vi "读取反控数据解析(子VI).vi"(6 "数据":string, 7 "命令编码CN":string) -> (0 "实时数据发送时间间隔/min":i32=1, 2 "设置超时时间/min":i32=1, 3 "反控命令错误？":bool)   [LabVIEW 2016, in "数据传输系统.lvlib"]
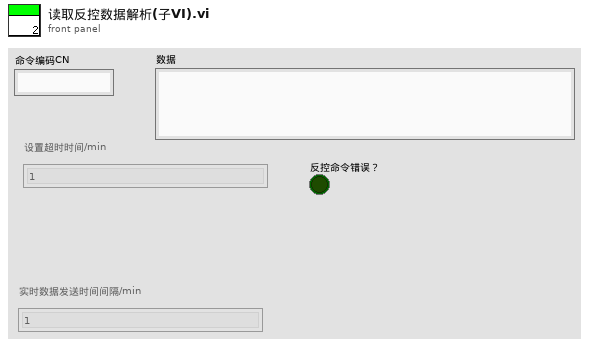
[diagram p1: front panel]
types:
  T1 = enum16{"初始化", "打开连接", "表格比对", "发送数据", "读取数据", "数据处理"}
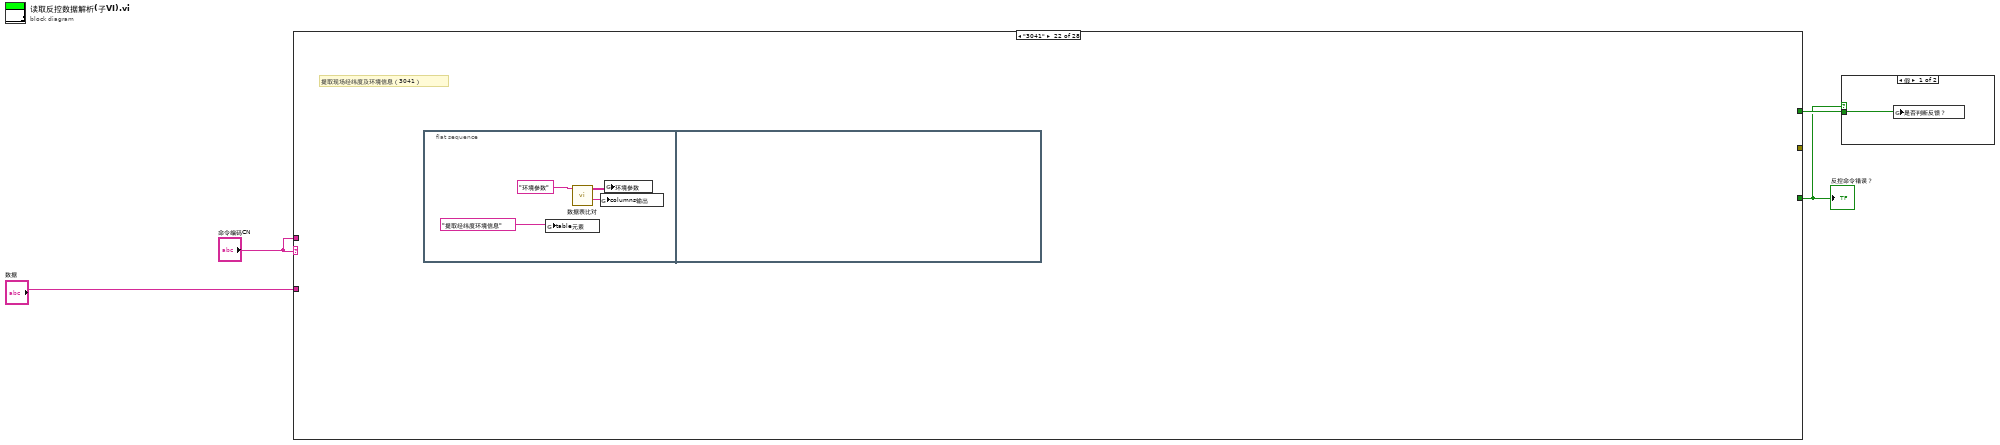
[diagram p0: block diagram]
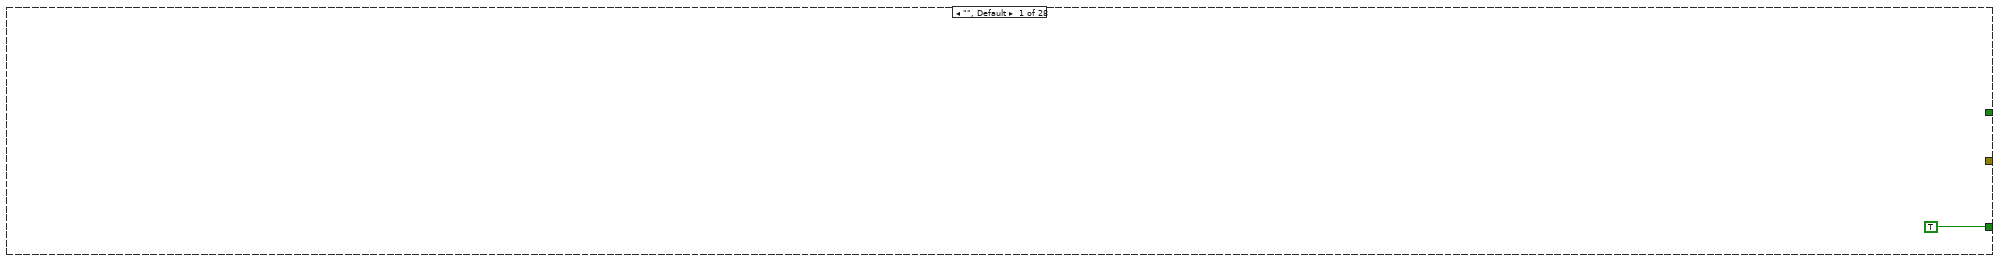
[diagram p3: hidden frame]
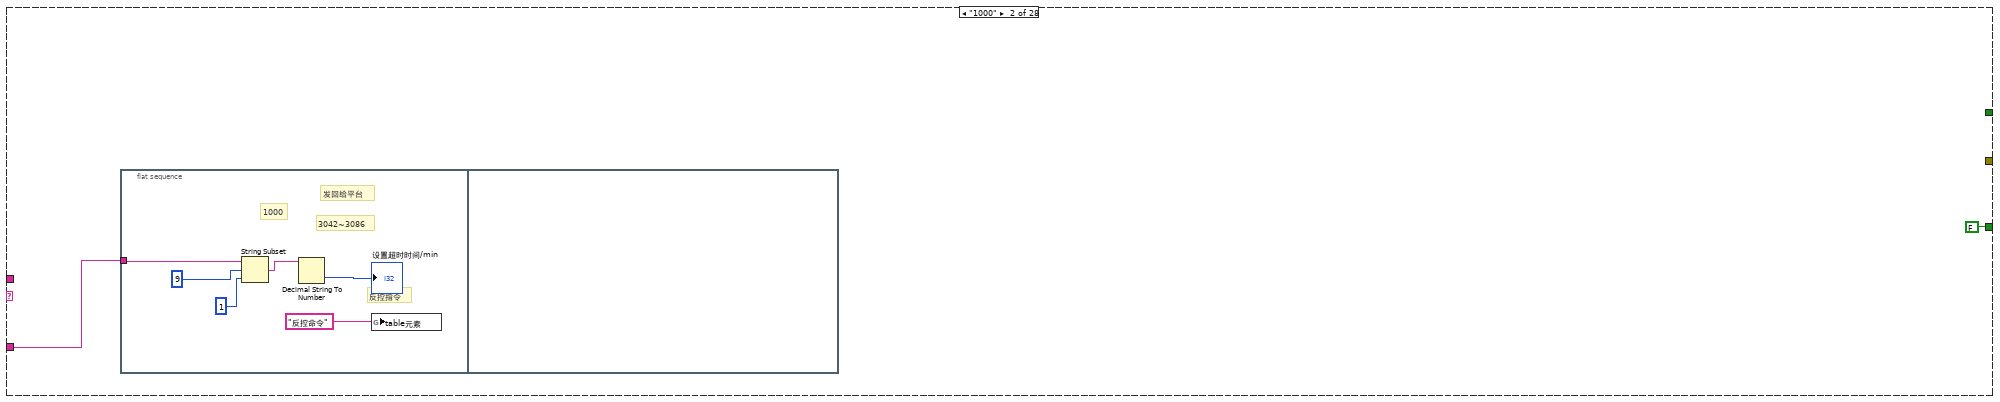
[diagram p4: hidden frame]
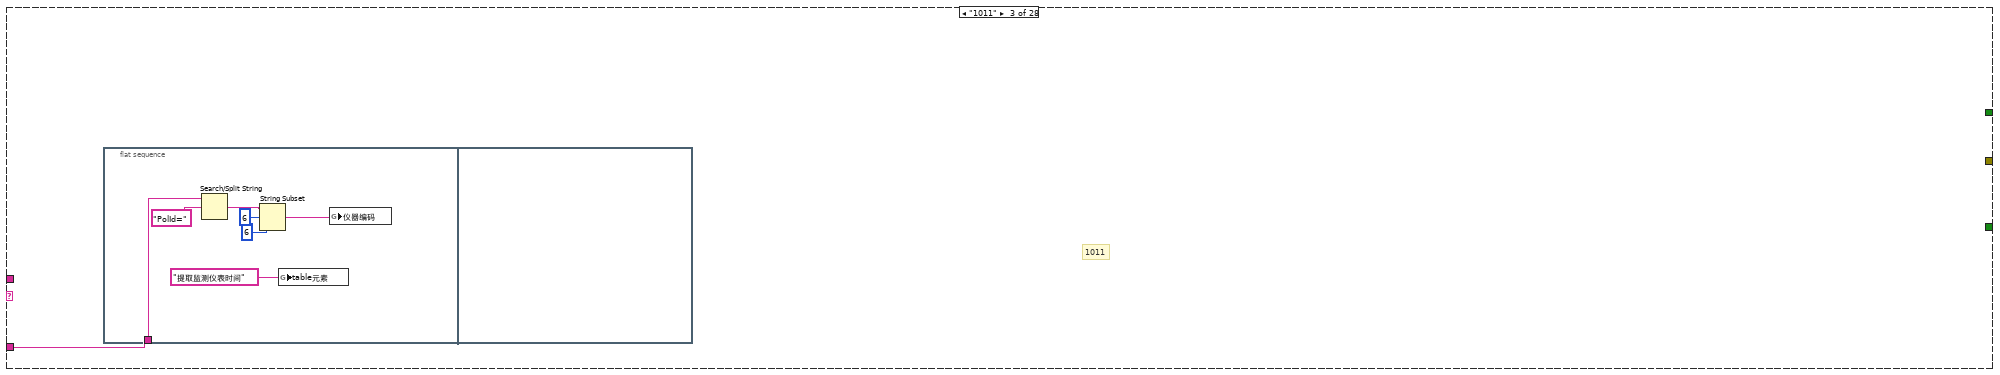
[diagram p5: hidden frame]
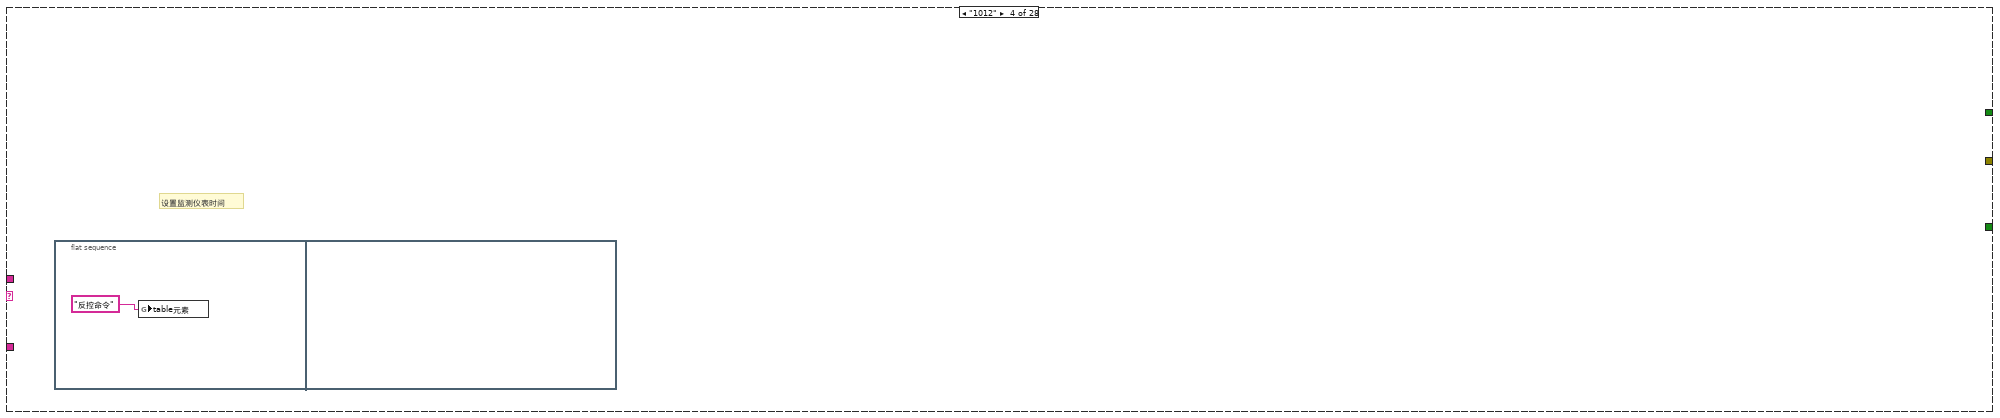
[diagram p6: hidden frame]
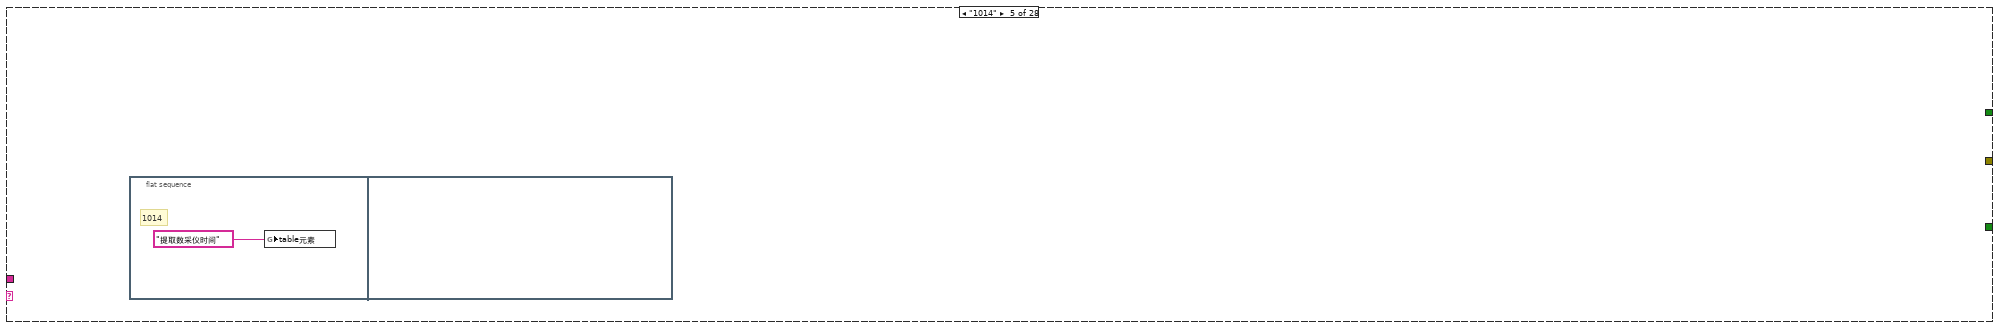
[diagram p7: hidden frame]
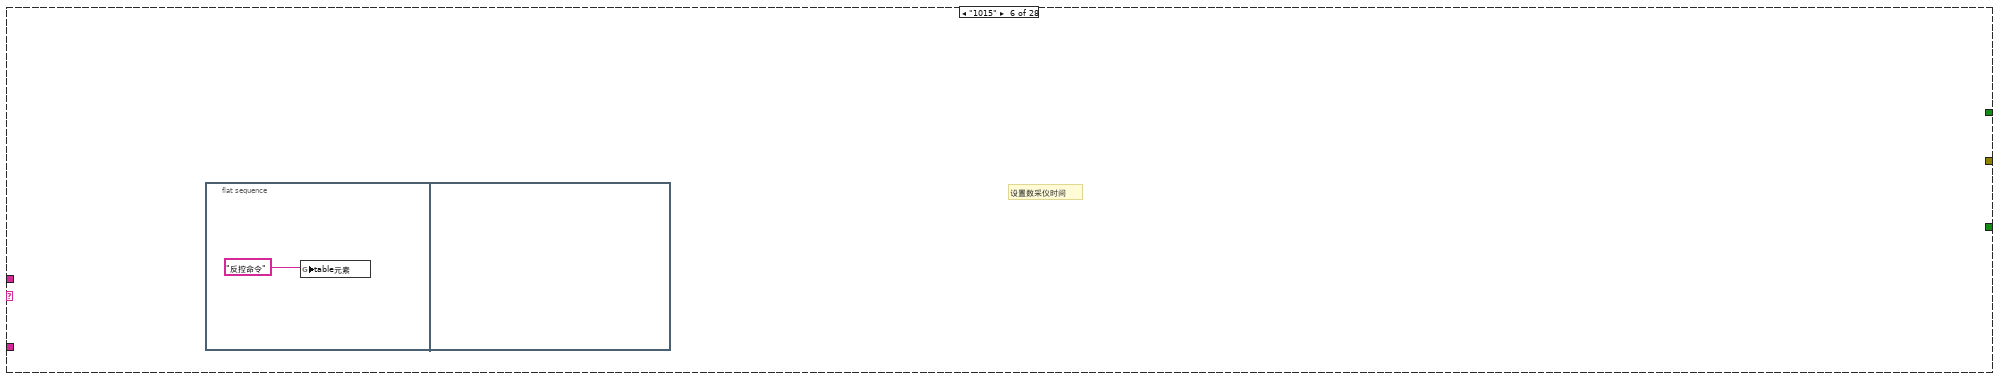
[diagram p8: hidden frame]
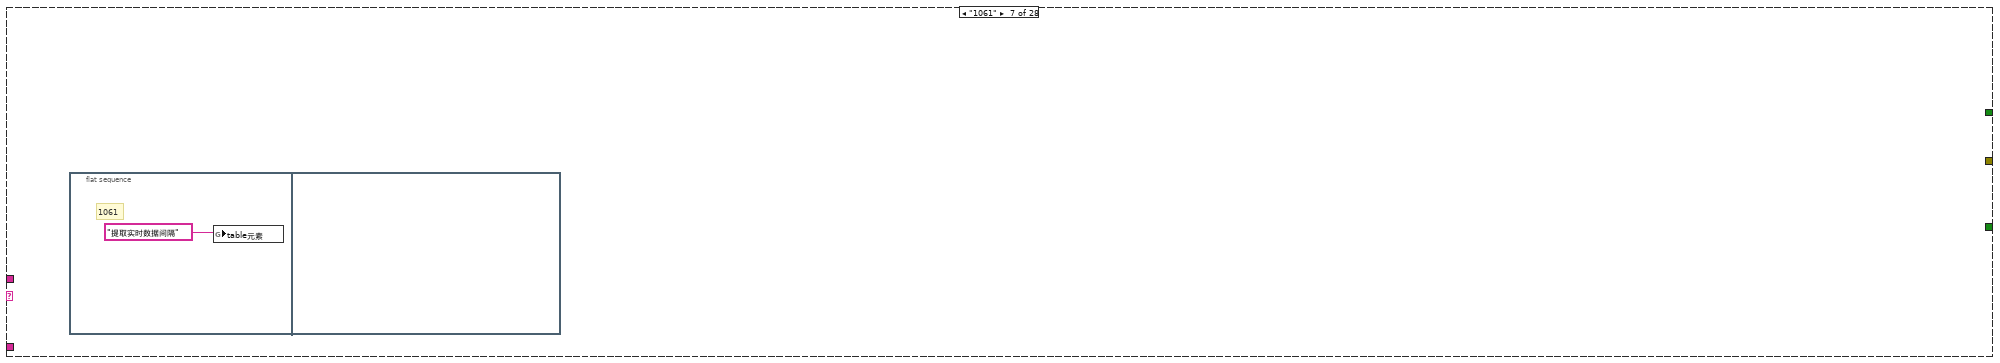
[diagram p9: hidden frame]
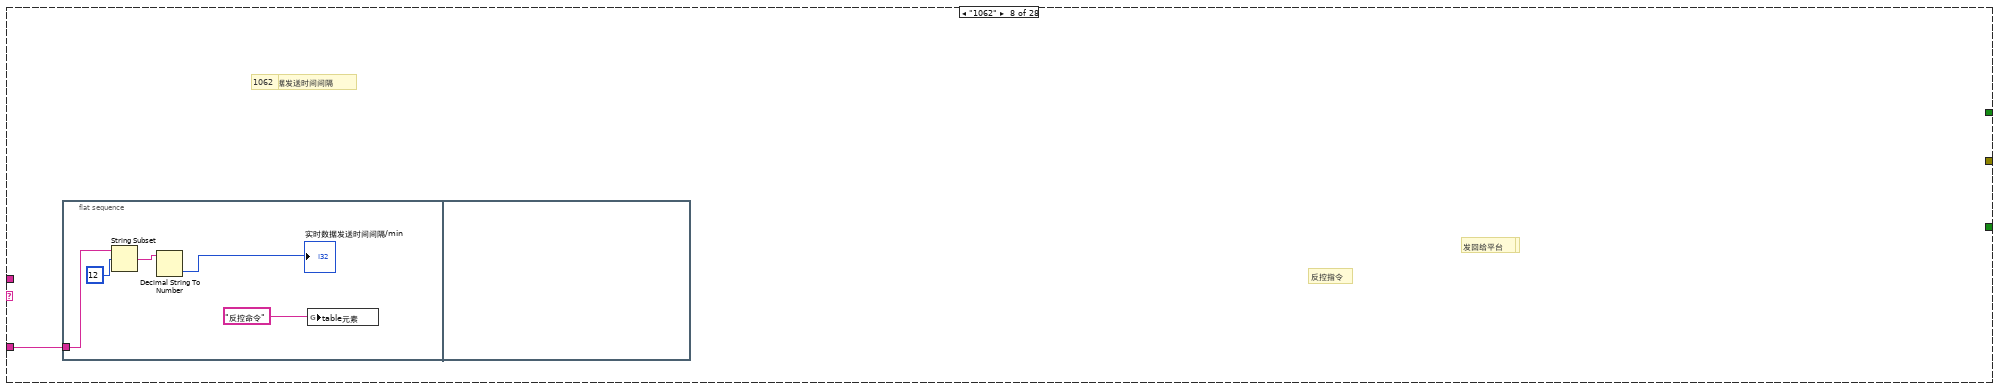
[diagram p10: hidden frame]
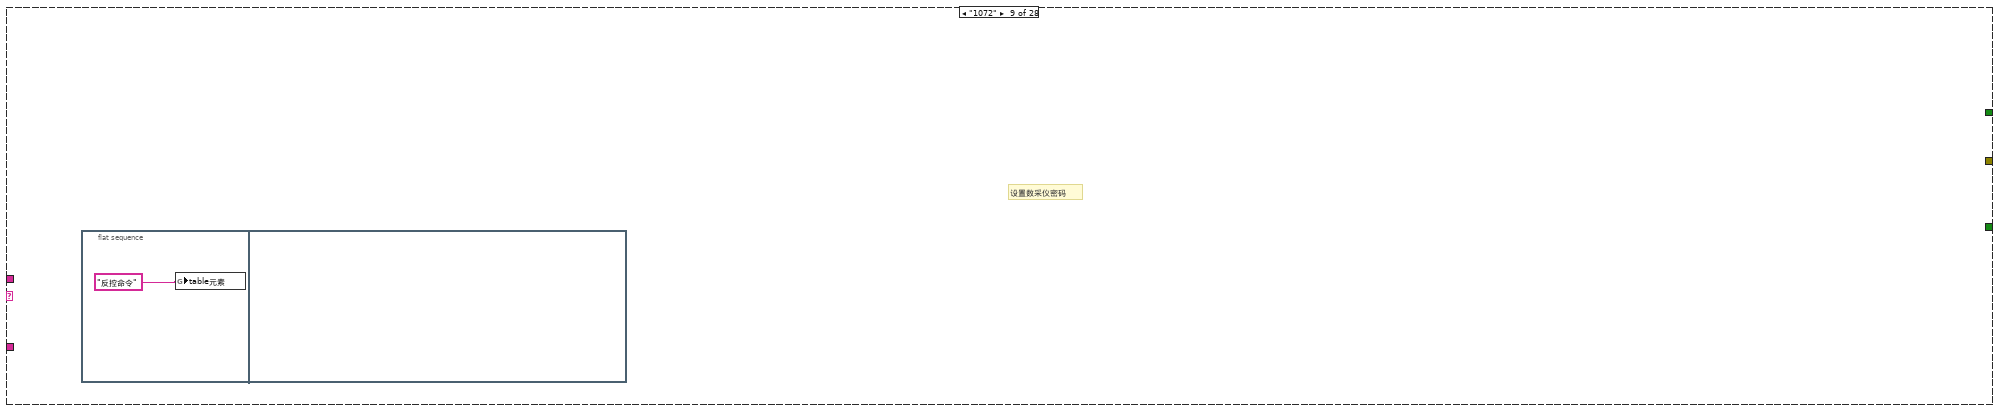
[diagram p11: hidden frame]
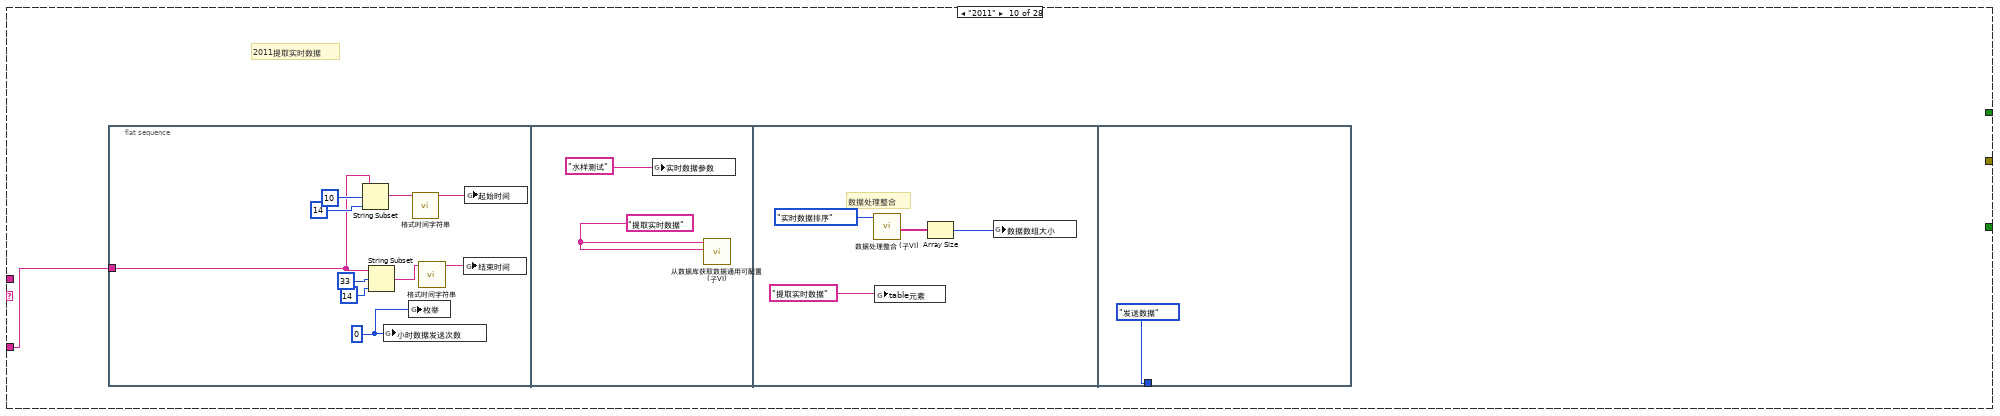
[diagram p12: hidden frame]
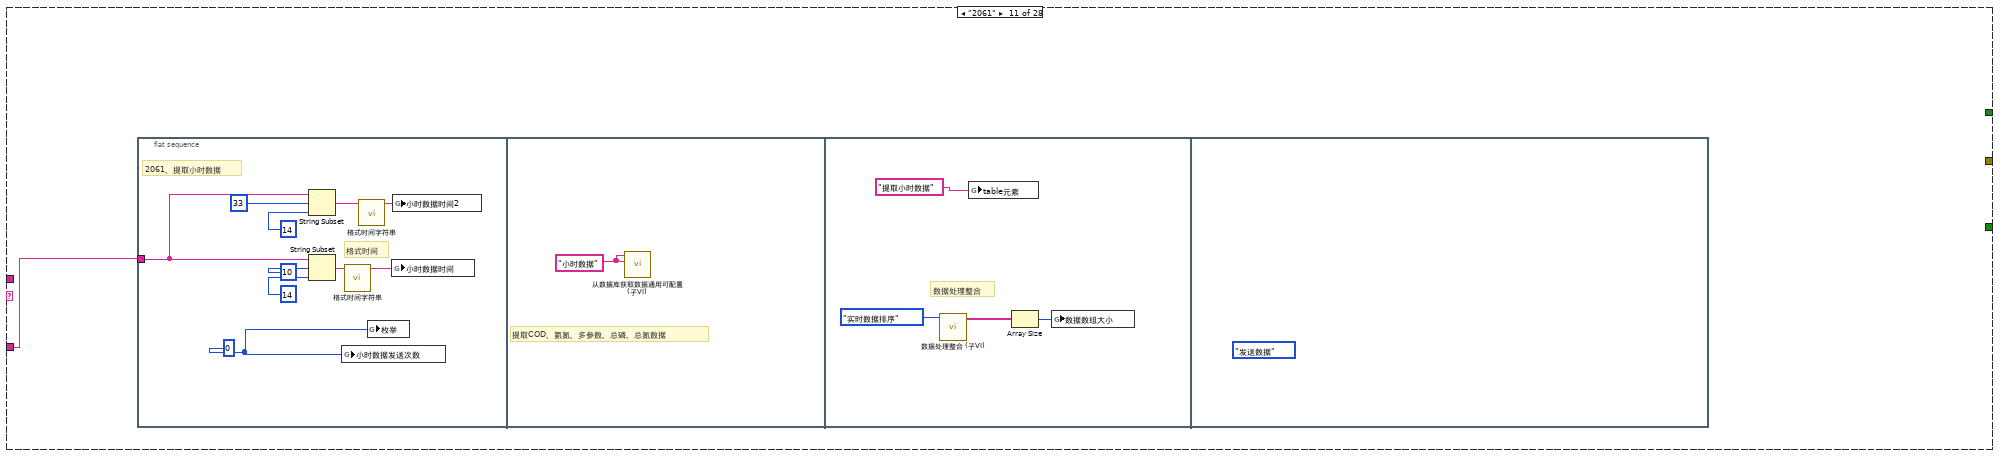
[diagram p13: hidden frame]
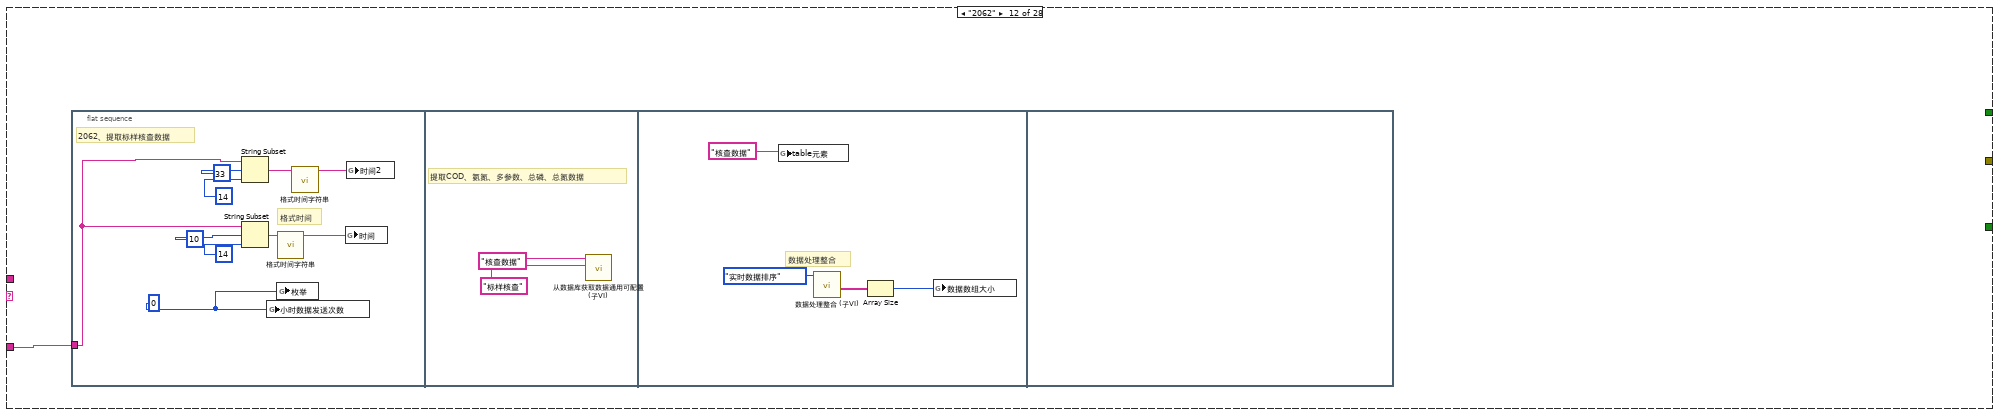
[diagram p14: hidden frame]
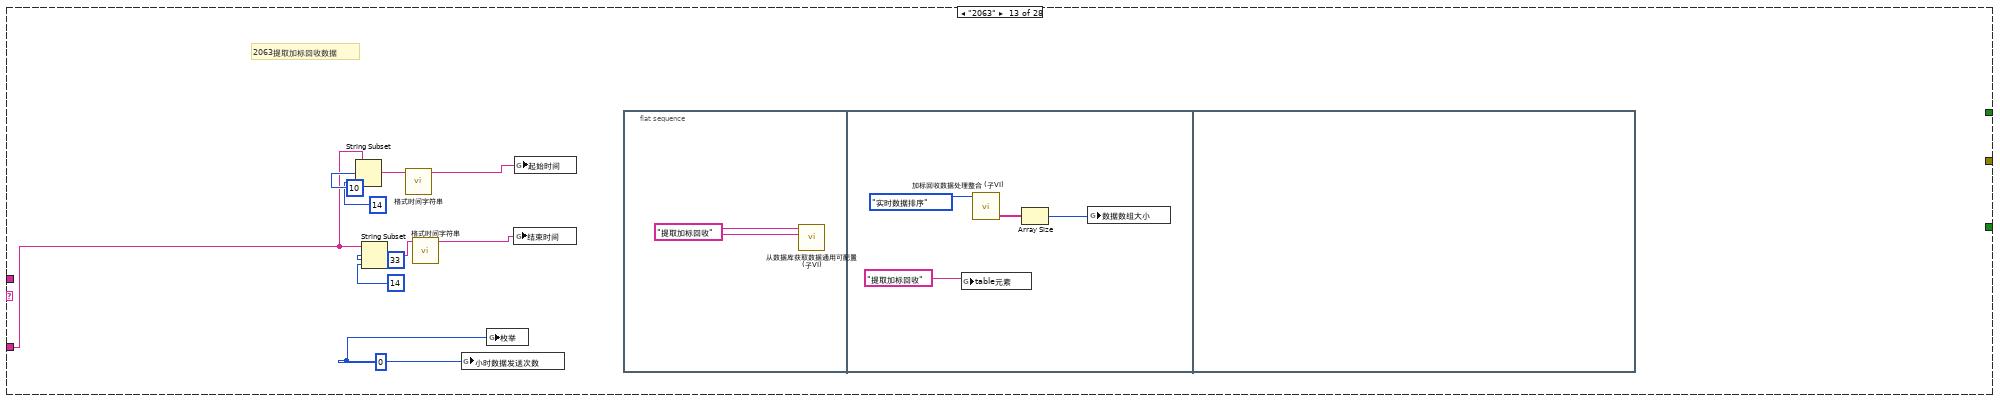
[diagram p15: hidden frame]
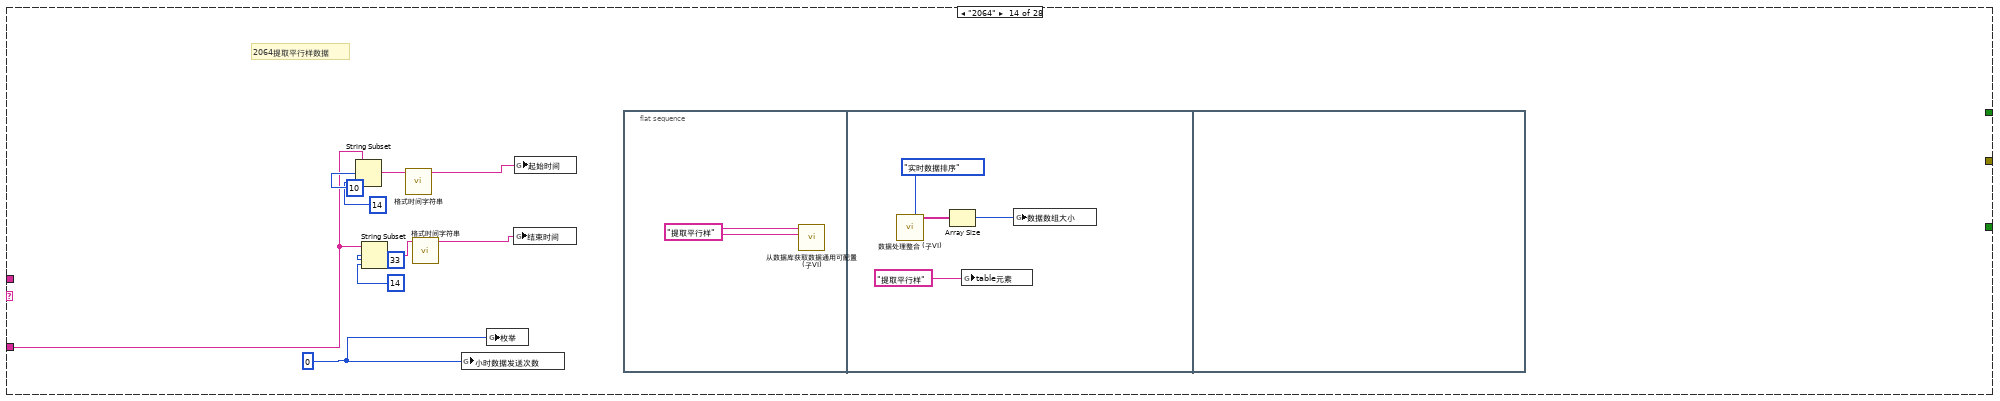
[diagram p16: hidden frame]
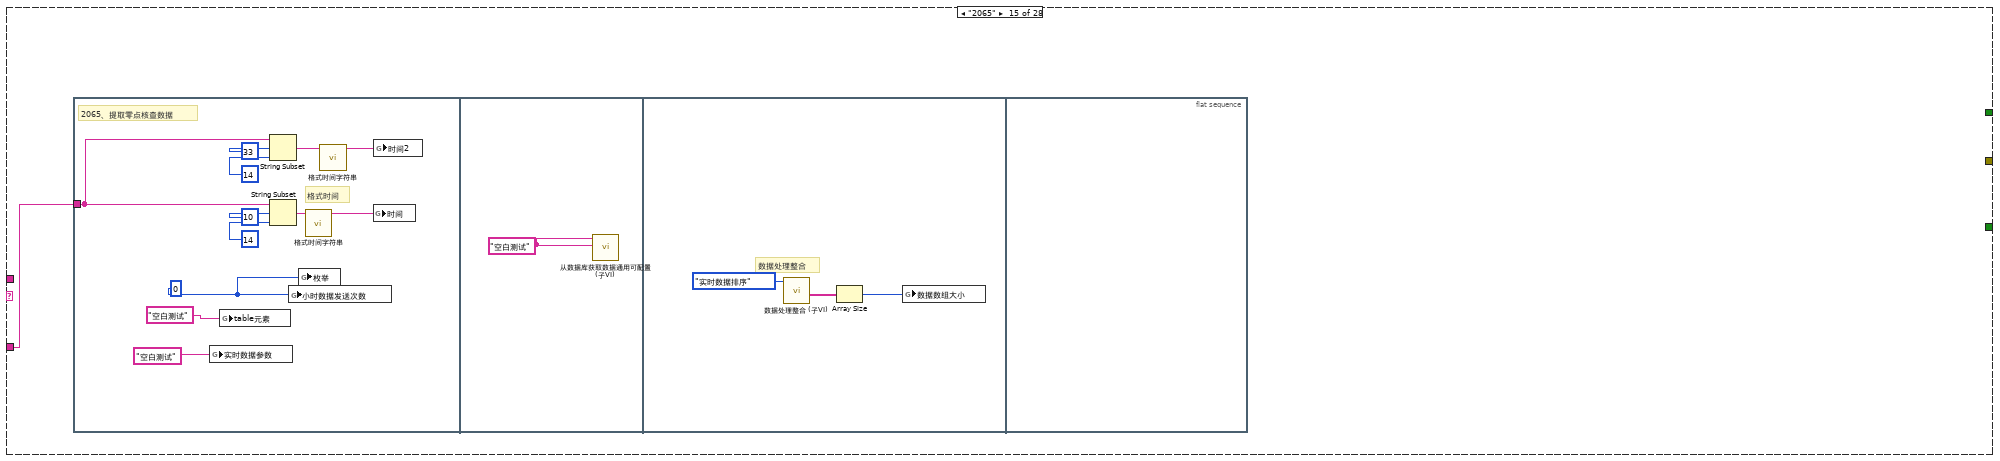
[diagram p17: hidden frame]
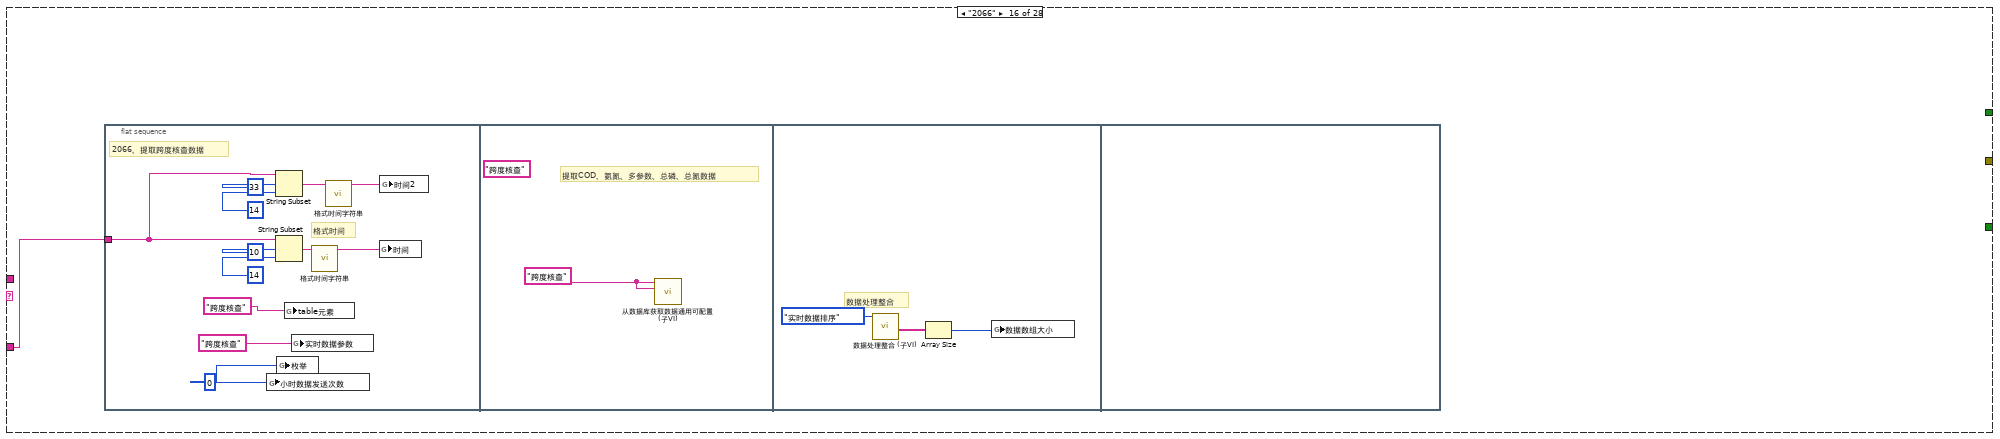
[diagram p18: hidden frame]
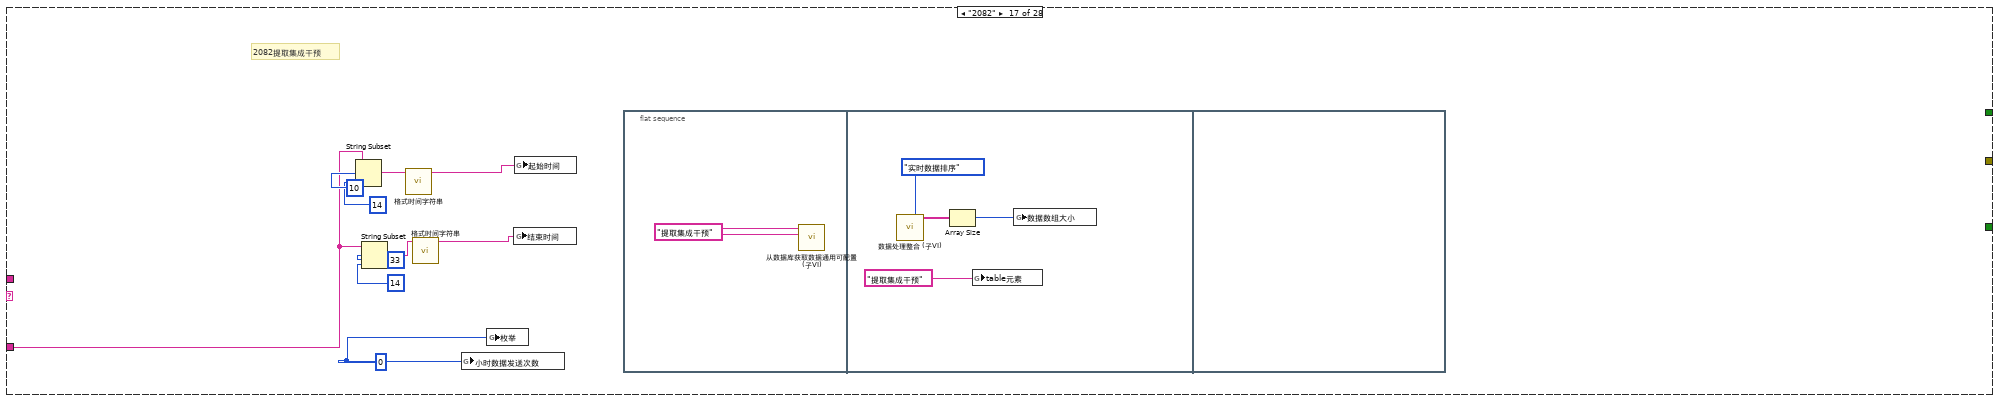
[diagram p19: hidden frame]
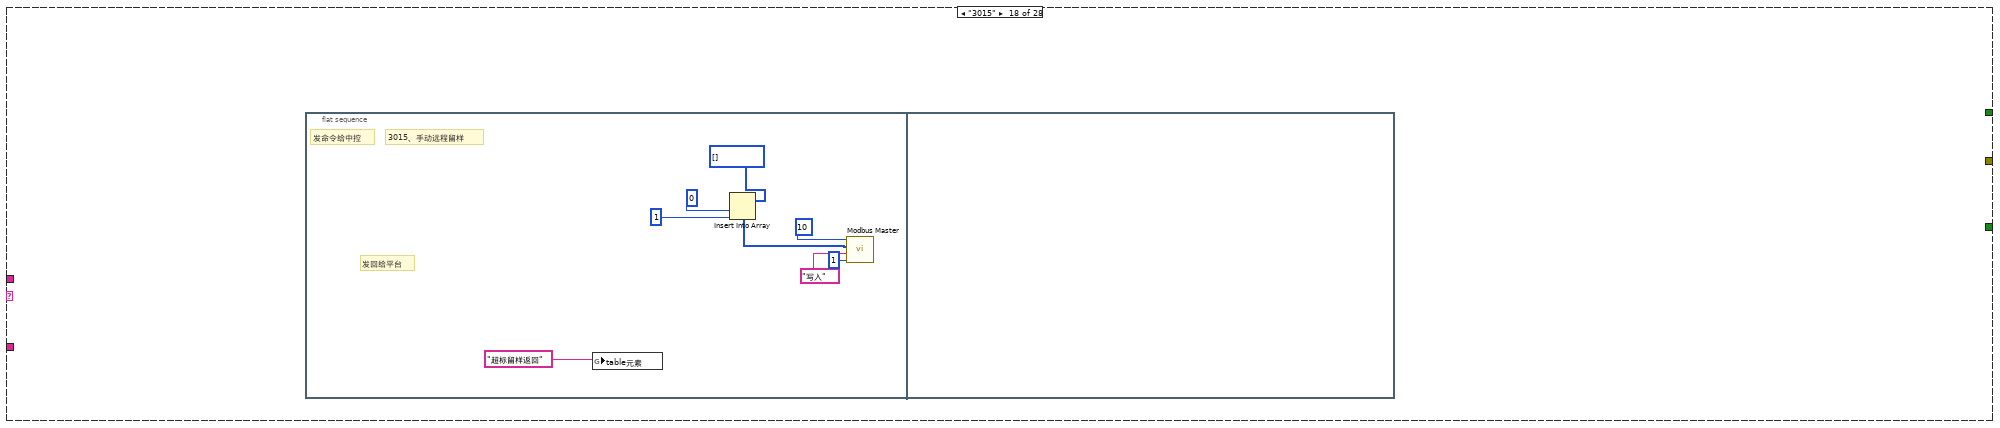
[diagram p20: hidden frame]
diagram:
  n1 = case shown="\"3041\"" "命令编码CN" {
    tunnel: "命令编码CN" -> [_ _ _ _ _ _ _ _ _ _ _ _ _ _ _ _ _ _ _ _ _ _ _ _ _ _ _ w469]
    tunnel: "数据" -> [_ w7 w14 _ _ _ _ w26 _ w33 w51 w67 w84 w99 w114 w131 w148 _ w174 w330 _ _ w408 _ _ _ w450 w466]
    tunnel: [_ _ _ _ _ _ _ _ _ _ _ _ _ _ _ _ _ _ _ _ _ _ _ _ _ _ _ w464] -> _
    tunnel: [TRUE FALSE _ _ _ _ _ _ _ _ _ _ _ _ _ _ _ _ _ _ _ _ _ _ _ _ _ _] -> w1
    tunnel: [_ _ _ _ _ _ _ _ _ _ _ _ _ _ _ _ _ _ FALSE ("是否判断反馈？") TRUE ("是否判断反馈？") _ _ TRUE ("是否判断反馈？") _ TRUE ("是否判断反馈？") TRUE ("是否判断反馈？") _ TRUE ("是否判断反馈？")] -> w2
    frame "", Default {
    }
    frame "1000" {
      n2 = flat-sequence {
        tunnel: w7 -> [w9]
        frame #0 {
          # "发回给平台"
          # "3042~3086"
          # "反控指令"
          # "1000"
          n3 = String Subset(string=w9, offset (0)=9 ("偏移量(0)"), length (rest)=1 ("长度（剩余）")) -> (substring=w11:string)
          n4 = Decimal String To Number(string=w11) -> (number=→"设置超时时间/min":i32)  [unwired: 2 in, 1 out]
          n5 = global write "全局1.vi" "table元素"("反控命令" ("新元素/子数组")) -> ()
        }
        frame #1 {
        }
      }
    }
    frame "1011" {
      # "1011"
      n6 = flat-sequence {
        tunnel: w14 -> [w16]
        frame #0 {
          n7 = Search/Split String(string=w16, search string/char (-)="PolId=" ("搜索字符串/字符(-)")) -> (match + rest of string=w20:string)  [unwired: 1 in, 2 out]
          n8 = String Subset(string=w20, offset (0)=6 ("偏移量(0)"), length (rest)=6 ("长度（剩余）")) -> (substring=w17:string)
          n9 = global write "全局1.vi" "table元素"("提取监测仪表时间") -> ()
          n10 = global write "全局 提取仪器参数.vi" "仪器编码"(w17) -> ()
        }
        frame #1 {
        }
      }
    }
    frame "1012" {
      # "设置监测仪表时间"
      n11 = flat-sequence {
        frame #0 {
          n12 = global write "全局1.vi" "table元素"("反控命令" ("新元素/子数组")) -> ()
        }
        frame #1 {
        }
      }
    }
    frame "1014" {
      n13 = flat-sequence {
        frame #0 {
          # "1014"
          n14 = global write "全局1.vi" "table元素"("提取数采仪时间") -> ()
        }
        frame #1 {
        }
      }
    }
    frame "1015" {
      # "设置数采仪时间"
      n15 = flat-sequence {
        frame #0 {
          n16 = global write "全局1.vi" "table元素"("反控命令" ("新元素/子数组")) -> ()
        }
        frame #1 {
        }
      }
    }
    frame "1061" {
      n17 = flat-sequence {
        frame #0 {
          # "1061"
          n18 = global write "全局1.vi" "table元素"("提取实时数据间隔") -> ()
        }
        frame #1 {
        }
      }
    }
    frame "1062" {
      # "发回给平台"
      # "反控指令"
      # "3042~3086"
      # "设置数据发送时间间隔"
      # "1062"
      n19 = flat-sequence {
        tunnel: w26 -> [w29]
        frame #0 {
          n20 = String Subset(string=w29, offset (0)=12 ("偏移量(0)")) -> (substring=w30:string)  [unwired: 1 in]
          n21 = Decimal String To Number(string=w30) -> (number=→"实时数据发送时间间隔/min":i32)  [unwired: 2 in, 1 out]
          n22 = global write "全局1.vi" "table元素"("反控命令" ("新元素/子数组")) -> ()
        }
        frame #1 {
        }
      }
    }
    frame "1072" {
      # "设置数采仪密码"
      n23 = flat-sequence {
        frame #0 {
          n24 = global write "全局1.vi" "table元素"("反控命令" ("新元素/子数组")) -> ()
        }
        frame #1 {
        }
      }
    }
    frame "2011" {
      # "2011提取实时数据"
      n25 = flat-sequence {
        tunnel: w33 -> [w34]
        tunnel: [T1."发送数据" ("元素")] -> _
        frame #0 {
          w39 = 0 ("数值")
          n26 = String Subset(string=w34, offset (0)=10 ("偏移量(0)"), length (rest)=14 ("长度（剩余）")) -> (substring=w42:string)
          n27 = String Subset(string=w34, offset (0)=33 ("偏移量(0)"), length (rest)=14 ("长度（剩余）")) -> (substring=w40:string)
          n28 = global write "全局 小时数据发送次数.vi" "小时数据发送次数"(w39) -> ()
          n29 = global write "全局1.vi" "枚举"(w39) -> ()
          n30 = call "格式时间字符串.vi"("字符串"=w42) -> ("连接的字符串"=w43:string)  [unwired: 10 in]
          n31 = call "格式时间字符串.vi"("字符串"=w40) -> ("连接的字符串"=w41:string)  [unwired: 10 in]
          n32 = global write "起始时间.vi" "结束时间"(w41) -> ()
          n33 = global write "起始时间.vi" "起始时间"(w43) -> ()
        }
        frame #1 {
          w44 = "提取实时数据" ("新元素/子数组")
          n34 = global write "全局 实时数据参数.vi" "实时数据参数"("水样测试") -> ()
          n35 = call "从数据库获取数据通用可配置(子VI).vi"("table输入"=w44, "列队名（唯一）"=w44) -> ()  [unwired: 8 in, 2 out]
        }
        frame #2 {
          # "数据处理整合"
          n36 = call "数据处理整合 (子VI).vi"("枚举"=enum16{"实时数据排序", "小时数据排序"}."实时数据排序") -> ("已排序的数组"=w48:string[])  [unwired: 10 in]
          n37 = global write "全局1.vi" "table元素"("提取实时数据" ("新元素/子数组")) -> ()
          n38 = Array Size(array=w48) -> (size(s)=w49:i32)
          n39 = global write "全局 数据数组大小.vi" "数据数组大小"(w49) -> ()
        }
        frame #3 {
        }
      }
    }
    frame "2061" {
      n40 = flat-sequence {
        tunnel: w51 -> [w52]
        frame #0 {
          w53 = 0 ("数值")
          # "格式时间"
          # "2061、提取小时数据"
          n41 = String Subset(string=w52, offset (0)=33 ("偏移量(0)"), length (rest)=14 ("长度（剩余）")) -> (substring=w55:string)
          n42 = String Subset(string=w52, offset (0)=10 ("偏移量(0)"), length (rest)=14 ("长度（剩余）")) -> (substring=w56:string)
          n43 = global write "全局 小时数据发送次数.vi" "小时数据发送次数"(w53) -> ()
          n44 = call "格式时间字符串.vi"("字符串"=w56) -> ("连接的字符串"=w57:string)  [unwired: 10 in]
          n45 = call "格式时间字符串.vi"("字符串"=w55) -> ("连接的字符串"=w54:string)  [unwired: 10 in]
          n46 = global write "全局1.vi" "枚举"(w53) -> ()
          n47 = global write "全局 水样时间.vi" "小时数据时间"(w57) -> ()
          n48 = global write "全局 时间2.vi" "小时数据时间2"(w54) -> ()
        }
        frame #1 {
          w62 = "小时数据" ("名称（未命名）")
          # "提取COD、氨氮、多参数、总磷、总氮数据"
          n49 = call "从数据库获取数据通用可配置(子VI).vi"("table输入"=w62, "列队名（唯一）"=w62) -> ()  [unwired: 8 in, 2 out]
        }
        frame #2 {
          # "数据处理整合"
          n50 = call "数据处理整合 (子VI).vi"("枚举"=enum16{"实时数据排序", "小时数据排序"}."实时数据排序") -> ("已排序的数组"=w66:string[])  [unwired: 10 in]
          n51 = global write "全局1.vi" "table元素"("提取小时数据" ("新元素/子数组")) -> ()
          n52 = Array Size(array=w66) -> (size(s)=w65:i32)
          n53 = global write "全局 数据数组大小.vi" "数据数组大小"(w65) -> ()
        }
        frame #3 {
          (unwired) T1."发送数据" ("元素")
        }
      }
    }
    frame "2062" {
      n54 = flat-sequence {
        tunnel: w67 -> [w68]
        frame #0 {
          w69 = 0 ("数值")
          # "格式时间"
          # "2062、提取标样核查数据"
          n55 = String Subset(string=w68, offset (0)=33 ("偏移量(0)"), length (rest)=14 ("长度（剩余）")) -> (substring=w71:string)
          n56 = String Subset(string=w68, offset (0)=10 ("偏移量(0)"), length (rest)=14 ("长度（剩余）")) -> (substring=w72:string)
          n57 = global write "全局 小时数据发送次数.vi" "小时数据发送次数"(w69) -> ()
          n58 = global write "全局1.vi" "枚举"(w69) -> ()
          n59 = call "格式时间字符串.vi"("字符串"=w72) -> ("连接的字符串"=w73:string)  [unwired: 10 in]
          n60 = call "格式时间字符串.vi"("字符串"=w71) -> ("连接的字符串"=w70:string)  [unwired: 10 in]
          n61 = global write "全局 水样时间.vi" "时间"(w73) -> ()
          n62 = global write "全局 时间2.vi" "时间2"(w70) -> ()
        }
        frame #1 {
          # "提取COD、氨氮、多参数、总磷、总氮数据"
          n63 = call "从数据库获取数据通用可配置(子VI).vi"("table输入"="标样核查" ("新元素/子数组"), "列队名（唯一）"="核查数据" ("新元素/子数组")) -> ()  [unwired: 8 in, 2 out]
        }
        frame #2 {
          # "数据处理整合"
          n64 = global write "全局1.vi" "table元素"("核查数据" ("新元素/子数组")) -> ()
          n65 = call "数据处理整合 (子VI).vi"("枚举"=enum16{"实时数据排序", "小时数据排序"}."实时数据排序") -> ("已排序的数组"=w82:string[])  [unwired: 10 in]
          n66 = Array Size(array=w82) -> (size(s)=w83:i32)
          n67 = global write "全局 数据数组大小.vi" "数据数组大小"(w83) -> ()
        }
        frame #3 {
        }
      }
    }
    frame "2063" {
      w89 = 0 ("数值")
      # "2063提取加标回收数据"
      n68 = String Subset(string=w84, offset (0)=10 ("偏移量(0)"), length (rest)=14 ("长度（剩余）")) -> (substring=w86:string)
      n69 = String Subset(string=w84, offset (0)=33 ("偏移量(0)"), length (rest)=14 ("长度（剩余）")) -> (substring=w88:string)
      n70 = call "格式时间字符串.vi"("字符串"=w86) -> ("连接的字符串"=w85:string)  [unwired: 10 in]
      n71 = call "格式时间字符串.vi"("字符串"=w88) -> ("连接的字符串"=w87:string)  [unwired: 10 in]
      n72 = global write "全局 小时数据发送次数.vi" "小时数据发送次数"(w89) -> ()
      n73 = global write "全局1.vi" "枚举"(w89) -> ()
      n74 = global write "起始时间.vi" "结束时间"(w87) -> ()
      n75 = global write "起始时间.vi" "起始时间"(w85) -> ()
      n76 = flat-sequence {
        frame #0 {
          w94 = "提取加标回收" ("新元素/子数组")
          n77 = call "从数据库获取数据通用可配置(子VI).vi"("table输入"=w94, "列队名（唯一）"=w94) -> ()  [unwired: 8 in, 2 out]
        }
        frame #1 {
          n78 = global write "全局1.vi" "table元素"("提取加标回收" ("新元素/子数组")) -> ()
          n79 = call "加标回收数据处理整合 (子VI).vi"("枚举"=enum16{"实时数据排序", "小时数据排序"}."实时数据排序") -> ("已排序的数组"=w96:string[])  [unwired: 10 in]
          n80 = Array Size(array=w96) -> (size(s)=w98:i32)
          n81 = global write "全局 数据数组大小.vi" "数据数组大小"(w98) -> ()
        }
        frame #2 {
        }
      }
    }
    frame "2064" {
      w104 = 0 ("数值")
      # "2064提取平行样数据"
      n82 = String Subset(string=w99, offset (0)=10 ("偏移量(0)"), length (rest)=14 ("长度（剩余）")) -> (substring=w101:string)
      n83 = String Subset(string=w99, offset (0)=33 ("偏移量(0)"), length (rest)=14 ("长度（剩余）")) -> (substring=w103:string)
      n84 = call "格式时间字符串.vi"("字符串"=w101) -> ("连接的字符串"=w100:string)  [unwired: 10 in]
      n85 = call "格式时间字符串.vi"("字符串"=w103) -> ("连接的字符串"=w102:string)  [unwired: 10 in]
      n86 = global write "全局 小时数据发送次数.vi" "小时数据发送次数"(w104) -> ()
      n87 = global write "全局1.vi" "枚举"(w104) -> ()
      n88 = global write "起始时间.vi" "结束时间"(w102) -> ()
      n89 = global write "起始时间.vi" "起始时间"(w100) -> ()
      n90 = flat-sequence {
        frame #0 {
          w109 = "提取平行样" ("新元素/子数组")
          n91 = call "从数据库获取数据通用可配置(子VI).vi"("table输入"=w109, "列队名（唯一）"=w109) -> ()  [unwired: 8 in, 2 out]
        }
        frame #1 {
          n92 = call "数据处理整合 (子VI).vi"("枚举"=enum16{"实时数据排序", "小时数据排序"}."实时数据排序") -> ("已排序的数组"=w113:string[])  [unwired: 10 in]
          n93 = Array Size(array=w113) -> (size(s)=w112:i32)
          n94 = global write "全局1.vi" "table元素"("提取平行样" ("新元素/子数组")) -> ()
          n95 = global write "全局 数据数组大小.vi" "数据数组大小"(w112) -> ()
        }
        frame #2 {
        }
      }
    }
    frame "2065" {
      n96 = flat-sequence {
        tunnel: w114 -> [w116]
        frame #0 {
          w117 = 0 ("数值")
          # "格式时间"
          # "2065、提取零点核查数据"
          n97 = global write "全局 实时数据参数.vi" "实时数据参数"("空白测试" ("新元素/子数组")) -> ()
          n98 = global write "全局1.vi" "table元素"("空白测试" ("新元素/子数组")) -> ()
          n99 = String Subset(string=w116, offset (0)=33 ("偏移量(0)"), length (rest)=14 ("长度（剩余）")) -> (substring=w120:string)
          n100 = String Subset(string=w116, offset (0)=10 ("偏移量(0)"), length (rest)=14 ("长度（剩余）")) -> (substring=w121:string)
          n101 = global write "全局 小时数据发送次数.vi" "小时数据发送次数"(w117) -> ()
          n102 = global write "全局1.vi" "枚举"(w117) -> ()
          n103 = call "格式时间字符串.vi"("字符串"=w121) -> ("连接的字符串"=w122:string)  [unwired: 10 in]
          n104 = call "格式时间字符串.vi"("字符串"=w120) -> ("连接的字符串"=w119:string)  [unwired: 10 in]
          n105 = global write "全局 水样时间.vi" "时间"(w122) -> ()
          n106 = global write "全局 时间2.vi" "时间2"(w119) -> ()
        }
        frame #1 {
          w127 = "空白测试" ("新元素/子数组")
          n107 = call "从数据库获取数据通用可配置(子VI).vi"("table输入"=w127, "列队名（唯一）"=w127) -> ()  [unwired: 8 in, 2 out]
        }
        frame #2 {
          # "数据处理整合"
          n108 = call "数据处理整合 (子VI).vi"("枚举"=enum16{"实时数据排序", "小时数据排序"}."实时数据排序") -> ("已排序的数组"=w129:string[])  [unwired: 10 in]
          n109 = Array Size(array=w129) -> (size(s)=w130:i32)
          n110 = global write "全局 数据数组大小.vi" "数据数组大小"(w130) -> ()
        }
        frame #3 {
        }
      }
    }
    frame "2066" {
      n111 = flat-sequence {
        tunnel: w131 -> [w133]
        frame #0 {
          w134 = 0 ("数值")
          # "格式时间"
          # "2066、提取跨度核查数据"
          n112 = global write "全局 小时数据发送次数.vi" "小时数据发送次数"(w134) -> ()
          n113 = String Subset(string=w133, offset (0)=33 ("偏移量(0)"), length (rest)=14 ("长度（剩余）")) -> (substring=w137:string)
          n114 = String Subset(string=w133, offset (0)=10 ("偏移量(0)"), length (rest)=14 ("长度（剩余）")) -> (substring=w138:string)
          n115 = global write "全局1.vi" "枚举"(w134) -> ()
          n116 = global write "全局1.vi" "table元素"("跨度核查" ("新元素/子数组")) -> ()
          n117 = global write "全局 实时数据参数.vi" "实时数据参数"("跨度核查" ("新元素/子数组")) -> ()
          n118 = call "格式时间字符串.vi"("字符串"=w138) -> ("连接的字符串"=w139:string)  [unwired: 10 in]
          n119 = call "格式时间字符串.vi"("字符串"=w137) -> ("连接的字符串"=w136:string)  [unwired: 10 in]
          n120 = global write "全局 水样时间.vi" "时间"(w139) -> ()
          n121 = global write "全局 时间2.vi" "时间2"(w136) -> ()
        }
        frame #1 {
          w144 = "跨度核查" ("新元素/子数组")
          (unwired) "跨度核查" ("名称（未命名）")
          # "提取COD、氨氮、多参数、总磷、总氮数据"
          n122 = call "从数据库获取数据通用可配置(子VI).vi"("table输入"=w144, "列队名（唯一）"=w144) -> ()  [unwired: 8 in, 2 out]
        }
        frame #2 {
          # "数据处理整合"
          n123 = call "数据处理整合 (子VI).vi"("枚举"=enum16{"实时数据排序", "小时数据排序"}."实时数据排序") -> ("已排序的数组"=w147:string[])  [unwired: 10 in]
          n124 = Array Size(array=w147) -> (size(s)=w146:i32)
          n125 = global write "全局 数据数组大小.vi" "数据数组大小"(w146) -> ()
        }
        frame #3 {
        }
      }
    }
    frame "2082" {
      w153 = 0 ("数值")
      # "2082提取集成干预"
      n126 = String Subset(string=w148, offset (0)=10 ("偏移量(0)"), length (rest)=14 ("长度（剩余）")) -> (substring=w150:string)
      n127 = String Subset(string=w148, offset (0)=33 ("偏移量(0)"), length (rest)=14 ("长度（剩余）")) -> (substring=w152:string)
      n128 = call "格式时间字符串.vi"("字符串"=w150) -> ("连接的字符串"=w149:string)  [unwired: 10 in]
      n129 = call "格式时间字符串.vi"("字符串"=w152) -> ("连接的字符串"=w151:string)  [unwired: 10 in]
      n130 = global write "全局 小时数据发送次数.vi" "小时数据发送次数"(w153) -> ()
      n131 = global write "全局1.vi" "枚举"(w153) -> ()
      n132 = global write "起始时间.vi" "结束时间"(w151) -> ()
      n133 = global write "起始时间.vi" "起始时间"(w149) -> ()
      n134 = flat-sequence {
        frame #0 {
          w158 = "提取集成干预" ("新元素/子数组")
          n135 = call "从数据库获取数据通用可配置(子VI).vi"("table输入"=w158, "列队名（唯一）"=w158) -> ()  [unwired: 8 in, 2 out]
        }
        frame #1 {
          n136 = call "数据处理整合 (子VI).vi"("枚举"=enum16{"实时数据排序", "小时数据排序"}."实时数据排序") -> ("已排序的数组"=w162:string[])  [unwired: 10 in]
          n137 = Array Size(array=w162) -> (size(s)=w161:i32)
          n138 = global write "全局1.vi" "table元素"("提取集成干预" ("新元素/子数组")) -> ()
          n139 = global write "全局 数据数组大小.vi" "数据数组大小"(w161) -> ()
        }
        frame #2 {
        }
      }
    }
    frame "3015" {
      n140 = flat-sequence {
        frame #0 {
          # "发命令给中控"
          # "发回给平台"
          # "3015、手动远程留样"
          n141 = global write "全局1.vi" "table元素"("超标留样返回" ("新元素/子数组")) -> ()
          n142 = Insert Into Array(array=u16[] [] ("holding register values"), index=0 ("索引"), new element=u16 1 ("新元素/子数组")) -> (w166:u16[])
          n143 = call "Modbus Master.vi"("Unit ID"=u8 1, "读取写入选择"="写入", "holding register values"=w166, "starting address"=u16 10) -> ()  [unwired: 6 in, 2 out]
        }
        frame #1 {
        }
      }
    }
    frame "3020" {
      n144 = flat-sequence {
        tunnel: [w184] -> w178
        tunnel: [w185] -> w177
        tunnel: [w181] -> w176
        tunnel: [w183] -> w175
        tunnel: w174 -> [w182]
        tunnel: [w182] -> w172
        tunnel: w178 -> [w217]
        tunnel: w177 -> [w216]
        tunnel: w176 -> [w215]
        tunnel: w175 -> [w214]
        tunnel: [w213] -> w173
        tunnel: w172 -> [w213]
        tunnel: w173 -> [w301]
        frame #0 {
          w179 = "操作日志报警信息" ("名称（未命名）")
          w188 = 0 ("数值")
          # "3020、提取日志、报警，仪器参数"
          n145 = Search/Split String(string=w182, search string/char (-)="BeginTime=" ("搜索字符串")) -> (match + rest of string=w187:string)  [unwired: 1 in, 2 out]
          n146 = call "日志报警参数选择 (子VI).vi"("String输入"=w182) -> ("输出boll数组"=w180:bool[], "输出char数组"=w181:string[])  [unwired: 7 in, 2 out]
          n147 = case shown="\"真\", 默认" w187 {
            tunnel: ["1904/01/01 00:00:00" w210] -> w190
            tunnel: w187 -> [_ w204]
            tunnel: [w198 w205] -> w186
            frame "" {
              n148 = Get Date/Time In Seconds() -> (seconds since 1Jan1904=w200:timestamp)
              n149 = Format Date/Time String(time format string (%c)="%Y/%m/%d %H:%M:%S" ("时间格式字符串(%c)"), seconds (now)=w200) -> (date/time string=w201:string)  [unwired: 1 in]
              n150 = Search and Replace String(input string=w201, search string="." ("搜索字符串")) -> (result string=w198:string)  [unwired: 6 in, 3 out]
            }
            frame "真", Default {
              # "格式时间"
              n151 = String Subset(string=w204, offset (0)=33 ("偏移量(0)"), length (rest)=14 ("长度（剩余）")) -> (substring=w208:string)
              n152 = String Subset(string=w204, offset (0)=10 ("偏移量(0)"), length (rest)=14 ("长度（剩余）")) -> (substring=w209:string)
              n153 = call "格式时间字符串.vi"("字符串"=w208) -> ("连接的字符串"=w205:string)  [unwired: 10 in]
              n154 = call "格式时间字符串.vi"("字符串"=w209) -> ("连接的字符串"=w210:string)  [unwired: 10 in]
            }
          }
          n155 = Or Array Elements(Boolean array=w180) -> (logical OR=w183:bool)
          n156 = global write "全局 水样时间.vi" "时间"(w190) -> ()
          n157 = global write "全局 时间2.vi" "时间2"(w186) -> ()
          n158 = global write "全局 小时数据发送次数.vi" "小时数据发送次数"(w188) -> ()
          n159 = Obtain Queue(name (unnamed)=w179, element data type=w179) -> (queue out=w184:refnum<queue>, error out=w185:errorcluster)  [unwired: 3 in, 1 out]
          n160 = case shown="真" w183 {
            tunnel: w184 -> [_ w192]
            tunnel: w180 -> [_ w191]
            frame False {
            }
            frame True {
              n161 = for {
                tunnel: w191 -> [w194] mode=indexing
                tunnel: w192 -> [w193]
                i -> [w195]
                n162 = case shown="真" w194 {
                  tunnel: w195 -> [_ w197]
                  tunnel: w193 -> [_ w196]
                  frame False {
                  }
                  frame True {
                    n163 = call "提取日志报警参数入列队 (子VI).vi"("索引"=w197, "队列输入"=w196) -> ()  [unwired: 10 in]
                  }
                }
              }
            }
          }
          n164 = global write "全局1.vi" "枚举"(w188) -> ()
        }
        frame #1 {
          # "按需求提取COD、氨氮、总磷、总氮日志"
          # "按需求提取COD、氨氮、总磷、总氮日志"
          n165 = case shown="真" w214 {
            tunnel: w216 -> [_ w220]
            tunnel: w217 -> [_ w219]
            tunnel: w215 -> [_ w218]
            frame False {
            }
            frame True {
              n166 = while {
                shift-right: [w221] -> _
                shift-left: w219 -> [w229]
                tunnel: w220 -> [w228]
                tunnel: w218 -> [w222]
                stop <- w225 stop-if-true
                n167 = Dequeue Element(queue=w229, error in (no error)=w228) -> (queue out=w227:refnum<queue>, element=w223:string)  [unwired: 1 in, 2 out]
                n168 = case shown="\"CODCr\"" w223 {
                  tunnel: w227 -> [_ _ _ _ _ _ _ _ _ _ _ _ _ _]
                  tunnel: w222 -> [w231 w236 w241 w246 w251 w257 w260 w265 w270 w275 w280 w285 w290 w295]
                  frame "CODMn", Default {
                    n169 = Index Array(array=w231, index=0 ("索引")) -> (element=w230:string)
                    n170 = call "数据表比对.vi"("仪器日志参数"="CODMn" ("元素"), "table输入"=w230) -> ("待发送数据"=w233:string[][])  [unwired: 6 in, 3 out]
                    n171 = global write "全局 所有参数.vi" "CODMn"(w233) -> ()
                  }
                  frame "CODCr" {
                    n172 = Index Array(array=w236, index=1 ("索引")) -> (element=w235:string)
                    n173 = call "数据表比对.vi"("仪器日志参数"="CODCr" ("元素"), "table输入"=w235) -> ("待发送数据"=w238:string[][])  [unwired: 6 in, 3 out]
                    n174 = global write "全局 所有参数.vi" "CODCr"(w238) -> ()
                  }
                  frame "氨氮" {
                    n175 = Index Array(array=w241, index=2 ("索引")) -> (element=w240:string)
                    n176 = call "数据表比对.vi"("仪器日志参数"="氨氮" ("元素"), "table输入"=w240) -> ("待发送数据"=w243:string[][])  [unwired: 6 in, 3 out]
                    n177 = global write "全局 所有参数.vi" "氨氮"(w243) -> ()
                  }
                  frame "总磷" {
                    n178 = Index Array(array=w246, index=3 ("索引")) -> (element=w245:string)
                    n179 = call "数据表比对.vi"("仪器日志参数"="总磷" ("元素"), "table输入"=w245) -> ("待发送数据"=w248:string[][])  [unwired: 6 in, 3 out]
                    n180 = global write "全局 所有参数.vi" "总磷"(w248) -> ()
                  }
                  frame "总氮" {
                    n181 = Index Array(array=w251, index=4 ("索引")) -> (element=w250:string)
                    n182 = call "数据表比对.vi"("仪器日志参数"="总氮" ("元素"), "table输入"=w250) -> ("待发送数据"=w253:string[][])  [unwired: 6 in, 3 out]
                    n183 = global write "全局 所有参数.vi" "总氮"(w253) -> ()
                  }
                  frame "数采仪" {
                    n184 = Index Array(array=w257, index=5 ("索引")) -> (element=w255:string)
                    n185 = call "数据表比对.vi"("仪器日志参数"="系统" ("元素"), "table输入"=w255) -> ("待发送数据"=w258:string[][])  [unwired: 6 in, 3 out]
                    n186 = global write "全局 所有参数.vi" "DO"(w258) -> ()
                  }
                  frame "PH" {
                    n187 = Index Array(array=w260, index=6 ("索引")) -> (element=w261:string)
                    n188 = call "数据表比对.vi"("仪器日志参数"="PH" ("元素"), "table输入"=w261) -> ("待发送数据"=w263:string[][])  [unwired: 6 in, 3 out]
                    n189 = global write "全局 所有参数.vi" "PH"(w263) -> ()
                  }
                  frame "电导率" {
                    n190 = Index Array(array=w265, index=7 ("索引")) -> (element=w266:string)
                    n191 = call "数据表比对.vi"("仪器日志参数"="电导率" ("元素"), "table输入"=w266) -> ("待发送数据"=w268:string[][])  [unwired: 6 in, 3 out]
                    n192 = global write "全局 所有参数.vi" "电导率"(w268) -> ()
                  }
                  frame "水温" {
                    n193 = Index Array(array=w270, index=8 ("索引")) -> (element=w271:string)
                    n194 = call "数据表比对.vi"("仪器日志参数"="水温" ("元素"), "table输入"=w271) -> ("待发送数据"=w273:string[][])  [unwired: 6 in, 3 out]
                    n195 = global write "全局 所有参数.vi" "水温"(w273) -> ()
                  }
                  frame "DO" {
                    n196 = Index Array(array=w275, index=9 ("索引")) -> (element=w276:string)
                    n197 = call "数据表比对.vi"("仪器日志参数"="溶解氧" ("元素"), "table输入"=w276) -> ("待发送数据"=w278:string[][])  [unwired: 6 in, 3 out]
                    n198 = global write "全局 所有参数.vi" "DO"(w278) -> ()
                  }
                  frame "浊度" {
                    n199 = Index Array(array=w280, index=10 ("索引")) -> (element=w281:string)
                    n200 = call "数据表比对.vi"("仪器日志参数"="浊度" ("元素"), "table输入"=w281) -> ("待发送数据"=w283:string[][])  [unwired: 6 in, 3 out]
                    n201 = global write "全局 所有参数.vi" "浊度"(w283) -> ()
                  }
                  frame "叶绿素" {
                    n202 = Index Array(array=w285, index=11 ("索引")) -> (element=w286:string)
                    n203 = call "数据表比对.vi"("仪器日志参数"="叶绿素" ("元素"), "table输入"=w286) -> ("待发送数据"=w288:string[][])  [unwired: 6 in, 3 out]
                    n204 = global write "全局 所有参数.vi" "叶绿素"(w288) -> ()
                  }
                  frame "藻密度" {
                    n205 = Index Array(array=w290, index=12 ("索引")) -> (element=w291:string)
                    n206 = call "数据表比对.vi"("仪器日志参数"="藻密度" ("元素"), "table输入"=w291) -> ("待发送数据"=w293:string[][])  [unwired: 6 in, 3 out]
                    n207 = global write "全局 所有参数.vi" "藻密度"(w293) -> ()
                  }
                  frame "ORP" {
                    n208 = Index Array(array=w295, index=13 ("索引")) -> (element=w296:string)
                    n209 = call "数据表比对.vi"("仪器日志参数"="ORP" ("元素"), "table输入"=w296) -> ("待发送数据"=w298:string[][])  [unwired: 6 in, 3 out]
                    n210 = global write "全局 所有参数.vi" "ORP"(w298) -> ()
                  }
                }
                n211 = Get Queue Status(queue=w227) -> (queue out=w221:refnum<queue>, # elements in queue=w226:i32)  [unwired: 2 in, 6 out]
                n212 = Wait (ms)(milliseconds to wait=u32 300 ("等待时间（毫秒）")) -> ()  [unwired: 1 out]
                n213 = Equal To 0?(x=w226) -> (x = 0?=w225:bool)
              }
            }
          }
        }
        frame #2 {
          w310 = "InfoId=" ("搜索字符串/字符(-)")
          n214 = Spreadsheet String To Array(delimiter (Tab)=";" ("分隔符(Tab)"), format string="" ("格式字符串"), spreadsheet string=w301, array type (2D Dbl)=string[] []) -> (array=w302:string[])
          n215 = Index Array(array=w302) -> (element=w300:string)  [unwired: 1 in]
          n216 = Search/Split String(string=w300, search string/char (-)=w310) -> (match + rest of string=w309:string)  [unwired: 1 in, 2 out]
          n217 = Search and Replace String(replace all?=TRUE ("替换全部？(F)"), input string=w309, search string=w310, replace string="" ("替换字符串(\"\")")) -> (result string=w306:string)  [unwired: 4 in, 3 out]
          n218 = Spreadsheet String To Array(delimiter (Tab)="," ("分隔符(Tab)"), format string="" ("格式字符串"), spreadsheet string=w306, array type (2D Dbl)=string[] []) -> (array=w308:string[])
          n219 = Index Array(array=w308) -> (element=w307:string)  [unwired: 1 in]
          n220 = case shown="\"i13001\", \"i13002\", \"i13003\", \"i13004\", \"i13005\", \"i13006\", \"i13007\", \"i13008\", \"i13009\", \"i13010\", \"i13011\", \"i13012\", \"i13013\", \"i13014\", \"i13015\", \"i13016\", \"i13017\", \"i13101\", \"i13102\", \"i13103\", \"i13104\", \"i13105\", \"i13106\", \"i13107\", \"i13108\", \"i13109\", \"i13110\"" w307 {
            tunnel: ["操作日志" ("名称（未命名）") "提取仪器参数" ("名称（未命名）") "报警信息" ("名称（未命名）") "" ("名称（未命名）")] -> w316
            tunnel: [w318 1 ("数据数组大小") 1 _] -> w317
            tunnel: w306 -> [_ w322 _ _]
            frame "i11001", "i21001" {
              # "数据处理整合"
              # "i11001日志"
              n221 = call "数据处理整合 (子VI).vi"("枚举"=enum16{"实时数据排序", "小时数据排序"}."实时数据排序") -> ("已排序的数组"=w319:string[])  [unwired: 10 in]
              n222 = Array Size(array=w319) -> (size(s)=w318:i32)
            }
            frame "i13001", "i13002", "i13003", "i13004", "i13005", "i13006", "i13007", "i13008", "i13009", "i13010", "i13011", "i13012", "i13013", "i13014", "i13015", "i13016", "i13017", "i13101", "i13102", "i13103", "i13104", "i13105", "i13106", "i13107", "i13108", "i13109", "i13110" {
              n223 = global write "全局 提取仪器参数.vi" "参数编码"(w322) -> ()
              n224 = call "数据处理直接插入整合 (子VI).vi"() -> ()  [unwired: 12 in]
            }
            frame "i12001" {
              # "i12001状态"
              n225 = call "数据处理直接插入整合 (子VI).vi"() -> ()  [unwired: 12 in]
            }
            frame Default {
            }
          }
          n226 = global write "全局 数据数组大小.vi" "数据数组大小"(w317) -> ()
          n227 = global write "全局1.vi" "table元素"(w316) -> ()
        }
      }
    }
    frame "3021" {
      (unwired) u16 256 ("starting address")
      (unwired) "PolId=w01018,InfoId=i13004,i13004-Info=168.0"
      # "0: 无\n1: CODMn\n2: PH\n3: 氨氮\n4: 总氮\n5: 总磷\n6:CODCr\n7:电导率\n8:水温\n9:溶解氧\n10:浊度\n11:叶绿素\n12:藻密度\n13:ORP"
      # "设置仪器参数"
      n228 = call "设置仪器参数命令解析.vi"("String输入"=w330) -> ("设置参数信息数组"=w329:string[][])  [unwired: 9 in, 1 out]
      n229 = for {
        tunnel: w329 -> [w333] mode=indexing
        # "同时设置几个参数?"
        n230 = flat-sequence {
          tunnel: w333 -> [w343]
          tunnel: [w334] -> w331
          tunnel: [w395] -> w332
          tunnel: w331 -> [w395]
          tunnel: w332 -> [w399]
          frame #0 {
            # "设置仪表参数"
            # "3|4个字节"
            # "反控指令"
            # "发命令给中控"
            # "1.因子编码\n2.关键参数\n3.值"
            n231 = Index Array(array=w343) -> (element #1=w342:string, element #2=w339:string, element #3=w338:string)  [unwired: 3 in]
            n232 = case shown="\"i13006\", \"i13013\"" w339 {
              tunnel: w338 -> [w347 w352]
              tunnel: [w345 w348] -> w336
              frame "假", Default {
                n233 = Fract/Exp String To Number(string=w347) -> (number=w344:dbl)  [unwired: 3 in, 1 out]
                n234 = Build Array(w344) -> (w346:dbl[])
                n235 = call "FloatToHex.vi"("浮点数"=w346) -> ("DCBA整形输出"=w345:u16[])  [unwired: 10 in]
              }
              frame "i13006", "i13013" {
                n236 = call "格式时间字符串.vi"("字符串"=w352) -> ("连接的字符串"=w351:string)  [unwired: 10 in]
                n237 = call "日期字符串格式至时间格式转换(子VI).vi"("data[0]"=w351) -> ("time stamp"=w350:timestamp)  [unwired: 10 in]
                n238 = Build Array(w350) -> (w349:timestamp[])
                n239 = call "DateToHex.vi"("DATE"=w349) -> ("数组"=w348:u16[])  [unwired: 10 in]
              }
            }
            n240 = case shown="\"w01100\"" w342 {
              tunnel: [u16 0 ("starting address") u16 1 ("starting address") u16 2 ("starting address") u16 3 ("starting address") u16 4 ("starting address") u16 5 ("starting address") u16 6 ("starting address") u16 7 ("starting address") u16 8 ("starting address") u16 9 ("starting address") u16 10 ("starting address") u16 11 ("starting address") u16 12 ("starting address") u16 13 ("starting address")] -> w337
              frame "", Default {
              }
              frame "w01019" {
              }
              frame "w01001" {
              }
              frame "w21003" {
              }
              frame "w21001" {
              }
              frame "w21011" {
              }
              frame "w01018" {
              }
              frame "w01014" {
              }
              frame "w01010" {
              }
              frame "w01009" {
              }
              frame "w01003" {
              }
              frame "w01016" {
              }
              frame "w19011" {
              }
              frame "w01100" {
              }
            }
            n241 = case shown="\"i13013\"" w339 {
              tunnel: [u16 256 ("starting address") u16 256 ("starting address") u16 260 ("starting address") u16 264 ("starting address") u16 268 ("starting address") u16 272 ("starting address") u16 276 ("starting address") u16 280 ("starting address") u16 284 ("starting address") u16 288 ("starting address") u16 292 ("starting address") u16 296 ("starting address") u16 300 ("starting address") u16 304 ("starting address") u16 308 ("starting address") u16 312 ("starting address") u16 316 ("starting address") u16 320 ("starting address") u16 356 ("starting address") u16 360 ("starting address") u16 364 ("starting address") u16 368 ("starting address") u16 372 ("starting address") u16 376 ("starting address") u16 380 ("starting address") u16 384 ("starting address") u16 388 ("starting address") u16 392 ("starting address")] -> w334
              frame "", Default {
              }
              frame "i13001" {
              }
              frame "i13002" {
              }
              frame "i13003" {
              }
              frame "i13004" {
              }
              frame "i13005" {
              }
              frame "i13006" {
              }
              frame "i13007" {
              }
              frame "i13008" {
              }
              frame "i13009" {
              }
              frame "i13010" {
              }
              frame "i13011" {
              }
              frame "i13012" {
              }
              frame "i13013" {
              }
              frame "i13014" {
              }
              frame "i13015" {
              }
              frame "i13016" {
              }
              frame "i13017" {
              }
              frame "i13101" {
              }
              frame "i13102" {
              }
              frame "i13103" {
              }
              frame "i13104" {
              }
              frame "i13105" {
              }
              frame "i13106" {
              }
              frame "i13107" {
              }
              frame "i13108" {
              }
              frame "i13109" {
              }
              frame "i13110" {
              }
            }
            n242 = Build Array (concatenate)(w337, w336) -> (w335:u16[])
            n243 = call "Modbus Master.vi"("Unit ID"=u8 1, "读取写入选择"="写入", "holding register values"=w335, "starting address"=w334) -> ()  [unwired: 6 in, 2 out]
          }
          frame #1 {
            n244 = Wait (ms)(milliseconds to wait=u32 3000 ("等待时间（毫秒）")) -> ()  [unwired: 1 out]
          }
          frame #2 {
            n245 = global write "全局1.vi" "table元素"("反控命令" ("新元素/子数组")) -> ()
            n246 = call "Modbus Master.vi"("Unit ID"=u8 1, "读取写入选择"="写入", "holding register values"=u16[] [0], "starting address"=w399) -> ()  [unwired: 6 in, 2 out]
          }
        }
      }
    }
    frame "3040" {
      # "提取现场系统信息（3040）"
      n247 = flat-sequence {
        frame #0 {
          n248 = global write "全局1.vi" "table元素"("提取现场系统信息" ("新元素/子数组")) -> ()
        }
        frame #1 {
        }
      }
    }
    frame "3041" {
      # "提取现场经纬度及环境信息（3041）"
      n249 = flat-sequence {
        frame #0 {
          n250 = global write "全局1.vi" "table元素"("提取经纬度环境信息" ("新元素/子数组")) -> ()
          n251 = call "数据表比对.vi"("table输入"="环境参数" ("新元素/子数组")) -> ("columns输出"=w403:string[], "待发送数据"=w405:string[][])  [unwired: 7 in, 2 out]
          n252 = global write "全局 环境参数.vi" "columns输出"(w403) -> ()
          n253 = global write "全局 环境参数.vi" "环境参数"(w405) -> ()
        }
        frame #1 {
        }
      }
    }
    frame "3042" {
      n254 = flat-sequence {
        tunnel: w408 -> [w410]
        frame #0 {
          # "反控指令"
          # "反控指令\n切换运行模式"
          # "发命令给中控"
          # "0维护，1常规，2应急，3质控"
          n255 = Search/Split String(string=w410, search string/char (-)="RunMode" ("搜索字符串/字符(-)")) -> (match + rest of string=w421:string)  [unwired: 1 in, 2 out]
          n256 = String Subset(string=w421, offset (0)=8 ("偏移量(0)"), length (rest)=1 ("长度（剩余）")) -> (substring=w418:string)
          n257 = case shown="\"0\", 默认" w418 {
            tunnel: [u16 0 ("新元素/子数组") u16 1 ("新元素/子数组") u16 2 ("新元素/子数组") u16 3 ("新元素/子数组")] -> w414
            frame "0", Default {
            }
            frame "1" {
            }
            frame "2" {
            }
            frame "3" {
            }
          }
          n258 = global write "全局1.vi" "table元素"("反控命令" ("新元素/子数组")) -> ()
          n259 = Insert Into Array(array=u16[] [] ("holding register values"), index=0 ("索引"), new element=w414) -> (w415:u16[])
          n260 = call "Modbus Master.vi"("Unit ID"=u8 1, "读取写入选择"="写入", "holding register values"=w415, "starting address"=u16 0) -> ()  [unwired: 6 in, 2 out]
        }
        frame #1 {
        }
      }
    }
    frame "3043" {
      # "远程重启工控机"
      n261 = flat-sequence {
        frame #0 {
          n262 = global write "全局1.vi" "table元素"("反控命令" ("新元素/子数组")) -> ()
        }
        frame #1 {
        }
      }
    }
    frame "3044" {
      n263 = flat-sequence {
        frame #0 {
          # "反控指令"
          # "发命令给中控"
          n264 = call "Modbus Master.vi"("Unit ID"=u8 1, "读取写入选择"="写入", "holding register values"=u16[] [1], "starting address"=u16 2) -> ()  [unwired: 6 in, 2 out]
        }
        frame #1 {
          # "反控指令\n单次测量"
          n265 = Wait (ms)(milliseconds to wait=u32 3000 ("等待时间（毫秒）")) -> ()  [unwired: 1 out]
        }
        frame #2 {
          n266 = global write "全局1.vi" "table元素"("反控命令" ("新元素/子数组")) -> ()
          n267 = call "Modbus Master.vi"("Unit ID"=u8 1, "读取写入选择"="写入", "holding register values"=u16[] [0], "starting address"=u16 2) -> ()  [unwired: 6 in, 2 out]
        }
      }
    }
    frame "3045", "3046" {
      n268 = flat-sequence {
        frame #0 {
          # "发命令给中控"
          n269 = call "Modbus Master.vi"("Unit ID"=u8 1, "读取写入选择"="写入", "holding register values"=u16[] [1], "starting address"=u16 3) -> ()  [unwired: 6 in, 2 out]
        }
        frame #1 {
          # "反控指令"
          # "反控指令\n急停"
          # "3045"
          n270 = Wait (ms)(milliseconds to wait=u32 3000 ("等待时间（毫秒）")) -> ()  [unwired: 1 out]
        }
        frame #2 {
          n271 = global write "全局1.vi" "table元素"("反控命令" ("新元素/子数组")) -> ()
          n272 = call "Modbus Master.vi"("Unit ID"=u8 1, "读取写入选择"="写入", "holding register values"=u16[] [0], "starting address"=u16 3) -> ()  [unwired: 6 in, 2 out]
        }
        frame #3 {
        }
      }
    }
    frame "3056" {
      n273 = flat-sequence {
        tunnel: w450 -> [w452]
        frame #0 {
          # "发回给平台"
          # "设置测量时间间隔"
          # "发命令给中控"
          n274 = Search/Split String(string=w452, search string/char (-)="RunInterval" ("搜索字符串/字符(-)")) -> (match + rest of string=w459:string)  [unwired: 1 in, 2 out]
          n275 = Decimal String To Number(string=w459, offset=12 ("偏移量(0)")) -> (number=w455:i32)  [unwired: 1 in, 1 out]
          n276 = Insert Into Array(array=u16[] [] ("holding register values"), index=0 ("索引"), new element=w455) -> (w454:u16[])
          n277 = global write "全局1.vi" "table元素"("反控命令" ("新元素/子数组")) -> ()
          n278 = call "Modbus Master.vi"("Unit ID"=u8 1, "读取写入选择"="写入", "holding register values"=w454, "starting address"=u16 14) -> ()  [unwired: 6 in, 2 out]
        }
        frame #1 {
        }
      }
    }
    frame "3080", "3081", "3082", "3083", "3084", "3085", "3086" {
      n279 = flat-sequence {
        tunnel: w469 -> [w473]
        tunnel: [w471] -> w468
        tunnel: w466 -> [w470]
        tunnel: w468 -> [w498]
        tunnel: [w498] -> w467
        tunnel: w467 -> [w503]
        tunnel: [w500] -> w465
        tunnel: [w506] -> w464
        tunnel: w465 -> [w506]
        frame #0 {
          # "30 启动标液核查  1CODmn  2 氨氮  3总磷  4总氮  5CODCr\n31 加标回收\n32 平行样测试\n33 零点核查\n34 跨度核查\n35 校零\n36 校标"
          # "1CODmn  2 氨氮  3总磷  4总氮  5CODCr"
          # "启动单台仪器标液核查"
          # "发命令给中控"
          n280 = Search/Split String(string=w470, search string/char (-)="PolId" ("搜索字符串/字符(-)")) -> (match + rest of string=w478:string)  [unwired: 1 in, 2 out]
          n281 = String Subset(string=w478, offset (0)=6 ("偏移量(0)"), length (rest)=6 ("长度（剩余）")) -> (substring=w475:string)
          n282 = case shown="\"w01019\"" w475 {
            tunnel: [0 ("长度（剩余）") 1 ("长度（剩余）") 2 ("长度（剩余）") 3 ("长度（剩余）") 4 ("长度（剩余）") 5 ("长度（剩余）")] -> w474
            frame "", Default {
            }
            frame "w01019" {
            }
            frame "w21003" {
            }
            frame "w21011" {
            }
            frame "w21001" {
            }
            frame "w01018" {
            }
          }
          n283 = Insert Into Array(array=u16[] [] ("holding register values"), index=0 ("索引"), new element=w474) -> (w479:u16[])
          n284 = case shown="\"3081\"" w473 {
            tunnel: [u16 99 ("starting address") u16 30 ("starting address") u16 31 ("starting address") u16 32 ("starting address") u16 33 ("starting address") u16 34 ("starting address") u16 35 ("starting address") u16 36 ("starting address")] -> w471
            frame "", Default {
            }
            frame "3080" {
            }
            frame "3081" {
            }
            frame "3082" {
            }
            frame "3083" {
            }
            frame "3084" {
            }
            frame "3085" {
            }
            frame "3086" {
            }
          }
          n285 = call "Modbus Master.vi"("Unit ID"=u8 1, "读取写入选择"="写入", "holding register values"=w479, "starting address"=w471) -> ()  [unwired: 6 in, 2 out]
        }
        frame #1 {
          n286 = Wait (ms)(milliseconds to wait=u32 3000 ("等待时间（毫秒）")) -> ()  [unwired: 1 out]
        }
        frame #2 {
          n287 = global write "全局1.vi" "table元素"("反控命令" ("新元素/子数组")) -> ()
          n288 = call "Modbus Master.vi"("Unit ID"=u8 1, "读取写入选择"="写入", "holding register values"=u16[] [0], "starting address"=w503) -> ("error out"=w500:errorcluster)  [unwired: 6 in, 1 out]
        }
        frame #3 {
        }
      }
    }
  }
  "反控命令错误？" <- w1
  n289 = case shown="假" w1 {
    tunnel: w2 -> [w507 _]
    frame False {
      n290 = global write "全局 反控命令枚举.vi" "是否判断反馈？"(w507) -> ()
    }
    frame True {
    }
  }
